vi "Untitled 6.vi"() -> ()   [LabVIEW 2018]
panel:
  out "Image Out":T1(plugin-control)
  in  "stop":bool
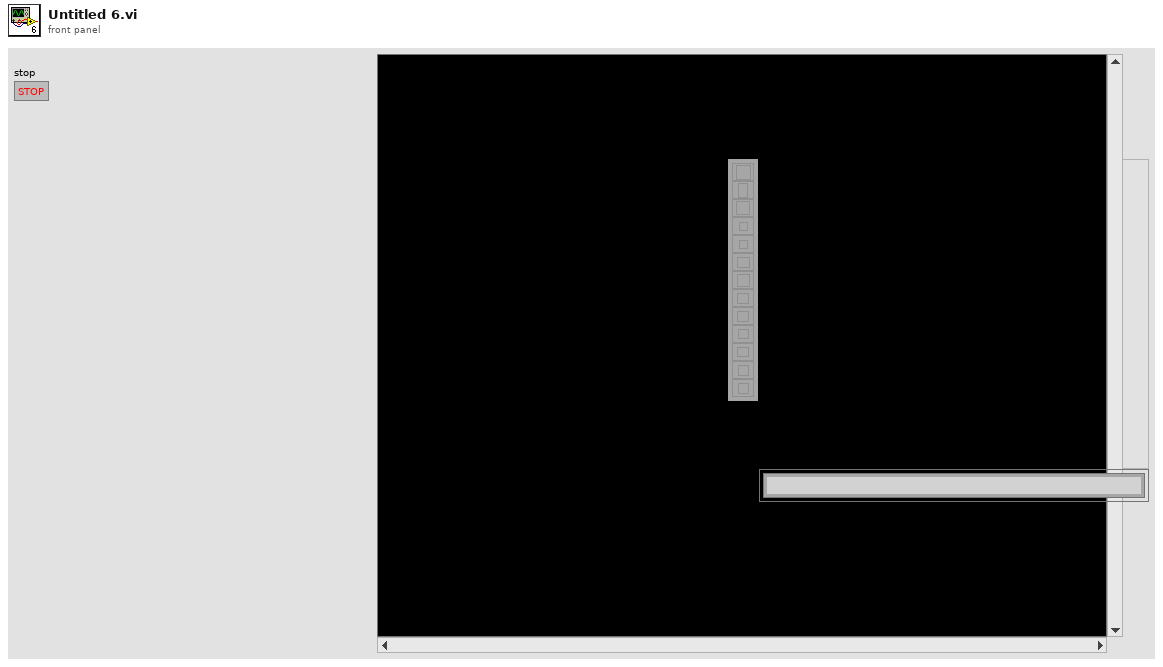
[diagram p1: front panel]
types:
  T1 = typedef "IMAQ Image.ctl" = refnum<image>
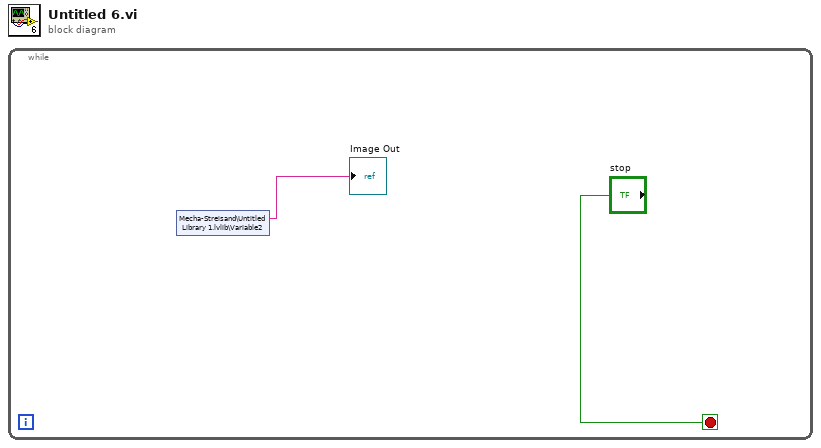
[diagram p0: block diagram]
diagram:
  n1 = while {
    stop <- "stop" stop-if-true
    n2 = shared-variable "Mecha-Streisand\\Untitled Library 1.lvlib\\Variable2"() -> (→"Image Out":string)  [unwired: 1 in, 1 out]
  }
